vi "GetLastErrorMessage.vi"(7 "DLL path":path, 8 "error in (no error)":errorcluster, 11 "session id in":i32) -> (0 "error out":errorcluster, 1 "LastErrorMessage":string, 3 "session id out":i32)   [LabVIEW 2017, in "ONNX Class Library.lvlib"]
doc: "/**\n * @brief Получить последнее сообщение об ошибке для сессии\n * \n * Возвращает детальное текстовое описание последней ошибки, произошедшей\n * при работе с сессией (загрузка, инференс и т.д.).\n * \n * @param sessionId [IN] ID сессии\n * @param buffer [OUT] Буфер для строки с сообщением об ошибке\n * @param bufferSize [IN] Размер буфера (рекомендуется 512 или больше)\n * \n * @return int32: 0 при успехе\n * @return int32: -1 если сессия не найдена\n * \n * @note Если ошибок не было, вернет \"No error\"\n * @note Сообщение сохраняется до вызова ClearLastError или DestroySession\n */\nint GetLastErrorMessage(int sessionId, char* buffer, int bufferSize);"
uses:
  ONNX Class Library.lvlib
panel:
  out "bufferSize":i32
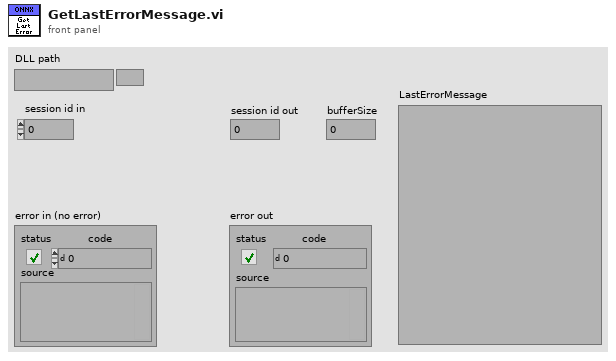
[diagram p1: front panel]
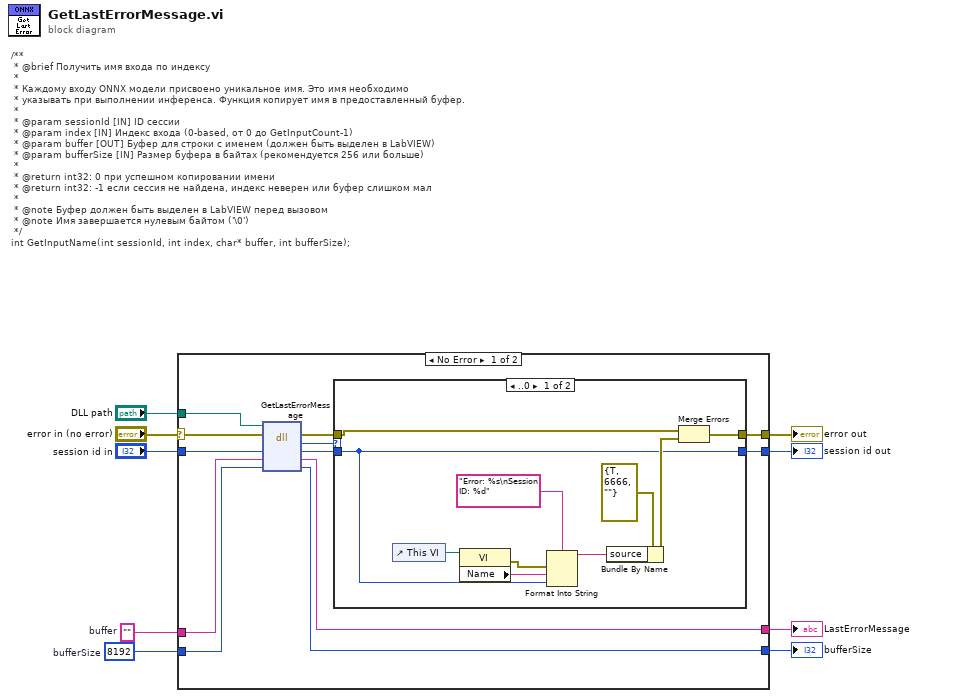
[diagram p0: block diagram]
diagram:
  w7 = 8192  # bufferSize
  w9 = ""  # buffer
  # "/**\n * @brief Получить имя входа по индексу\n * \n * Каждому входу ONNX модели присвоено уникальное имя. Это имя необходимо\n * указывать при выполнении инференса. Функция копирует имя в предоставленный буфер.\n * \n * @param sessionId [IN] ID сессии\n * @param index [IN] Индекс входа (0-based, от 0 до GetInputCount-1)\n * @param buffer [OUT] Буфер для строки с именем (должен быть выделен в LabVIEW)\n * @param bufferSize [IN] Размер буфера в байтах (рекомендуется 256 или больше)\n * \n * @return int32: 0 при успешном копировании имени\n * @return int32: -1 если сессия не найдена, индекс неверен или буфер слишком мал\n * \n * @note Буфер должен быть выделен в LabVIEW перед вызовом\n * @note Имя завершается нулевым байтом ('\\0')\n */\nint GetInputName(int sessionId, int index, char* buffer, int bufferSize);"
  n1 = case shown="No Error" "error in (no error)" {
    selector: "error in (no error)" -> [w10 w35]
    tunnel: w9 -> [w21 _]
    tunnel: [w20 _] -> w8
    tunnel: w7 -> [w19 _]
    tunnel: "session id in" -> [w18 w34]
    tunnel: [w17 _] -> w5
    tunnel: [w13 w35] -> w4
    tunnel: [w12 w34] -> w3
    tunnel: "DLL path" -> [w11 _]
    frame No Error {
      n2 = dll-call lib="home/ivan/LabVIEWData/ONNX/Test/libonnx_wrapper/unix64/libonnx_wrapper.so" fn="GetLastErrorMessage"(path in=w11, error in=w10, "sessionId"=w18, "buffer"=w21, "bufferSize"=w19) -> (error out=w16:errorcluster, "return"=w15:i32, "sessionId"=w14:i32, "buffer"=w20:string, "bufferSize"=w17:i32)  [unwired: 1 in, 1 out]
      n3 = case shown="..0" w15 {
        tunnel: w16 -> [w22 w33]
        tunnel: [w23 w33] -> w13
        tunnel: w14 -> [w24 w32]
        tunnel: [w24 w32] -> w12
        frame ..0 {
          n4 = control-ref of="This VI"() -> (w28:refnum<vi>)
          n5 = property class="VI"(reference=w28) -> (error out=w25:errorcluster, "Name"=w27:string)  [unwired: 1 in, 1 out]
          n6 = Format Into String(format string="Error: %s\nSession ID: %d", error in=w25, w27, w24) -> (resulting string=w29:string)  [unwired: 1 in, 1 out]
          n7 = Bundle By Name(cluster=errorcluster {"status"=TRUE, "code"=6666, "source"=""} ("error out"), "source"=w29) -> (w30:errorcluster)
          n8 = Merge Errors(w22, w30) -> (w23:errorcluster)
        }
        frame 1.. {
        }
      }
    }
    frame Error {
    }
  }
  "error out" <- w4
  "session id out" <- w3
  "LastErrorMessage" <- w8
  "bufferSize" <- w5
